vi "Abort Sequence Load.vi"() -> (1 "Abort Sequence":T1 {"Sequence Controller"."Valve" items=["None", "LOX Press", "LOX Purge", "LOX Vent", "LOX Iso", "LOX Main", "LOX Bleed", "*open*", "Fuel Press", "Fuel Purge", "Fuel Vent", "Fuel Iso", "Fuel Main", "Film Cooling", "*open*", "Ignition", "Trigger"]})   [LabVIEW 2024]
uses:
  Sequence Structure.ctl
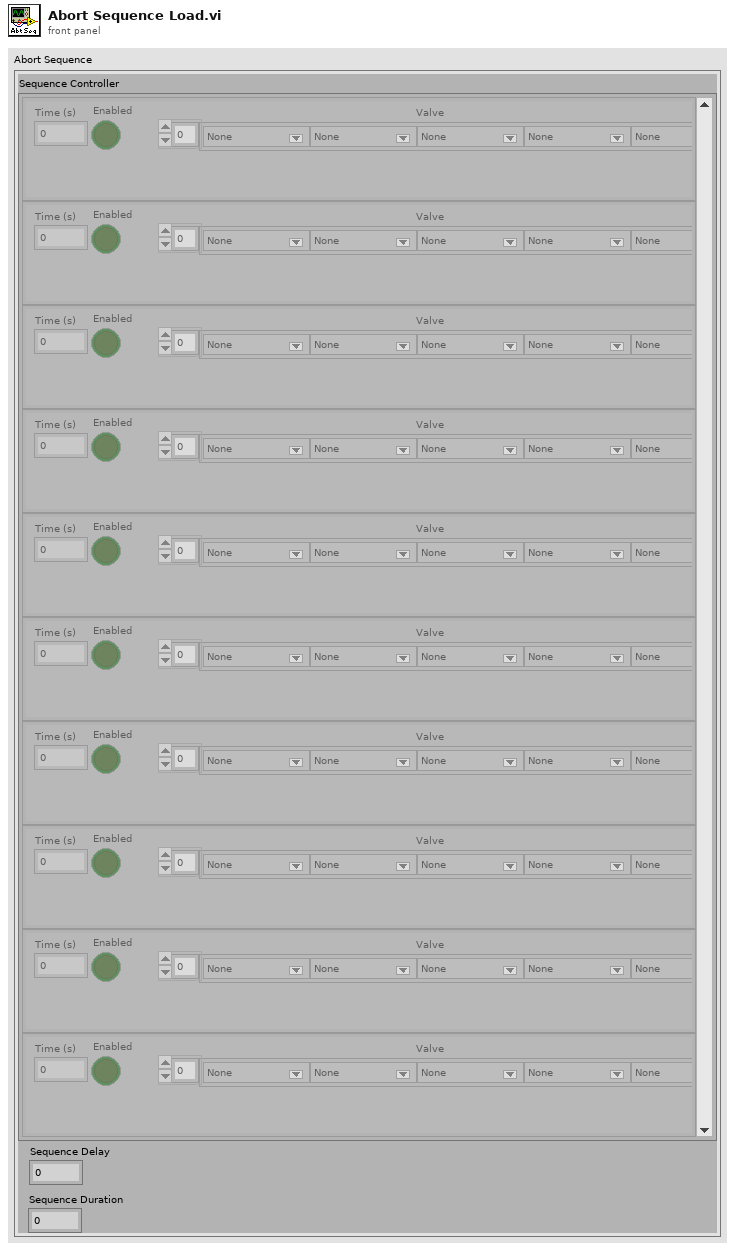
[diagram p1: front panel]
types:
  T1 = typedef "Sequence Structure.ctl" = cluster{"Sequence Controller":cluster{"Time (s)":dbl, "Enabled":bool, "Valve":u16[]}[], "Sequence Delay":dbl, "Sequence Duration":dbl}
  T2 = cluster{"Time (s)":dbl, "Enabled":bool, "Valve":u16[]}[]
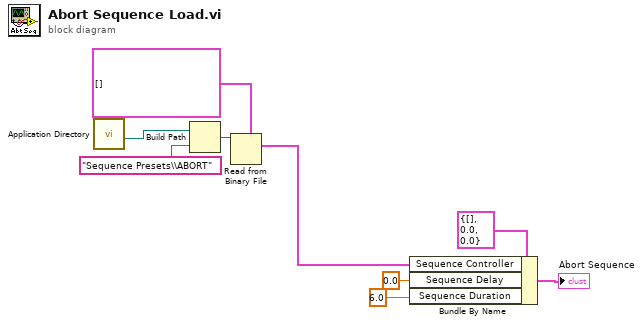
[diagram p0: block diagram]
diagram:
  n1 = call <vilib>:"Application Directory.vi"() -> ("Application Directory"=w6:path)
  n2 = Build Path(base path=w6, name or relative path="Sequence Presets\\ABORT") -> (appended path=w8:path)
  n3 = Read from Binary File(5:T2 [] ("Sequence Controller"), 11:w8) -> (2:w3:T2)  [unwired: 4 in, 3 out]
  n4 = Bundle By Name(cluster=T1 {"Sequence Controller"=[], "Sequence Delay"=0.0, "Sequence Duration"=0.0} ("Abort Sequence"), "Sequence Controller"=w3, "Sequence Delay"=0.0, "Sequence Duration"=6.0) -> (→"Abort Sequence":T1)
